vi "ao_waveform_full.vi"() -> ()   [LabVIEW 2020]
uses:
  <vilib>/measure/NI_MABase.lvlib
panel:
  in  "Offset":dbl
  in  "signal type":T1(ring) caption="Signal Type"
  out "error out":errorcluster caption="错误输出"
  in  "Frequency":dbl=1000.0 format="%#.6g"
  in  "Amplitude":dbl=5.0 format="%.3f"
  out "波形图":waveform(dbl)(graph)
  in  "AoCycle":u32
  in  "SamplePeriod(ns)":u32=10000
  in  "Chan":u8
  in  "DevIndex":i32
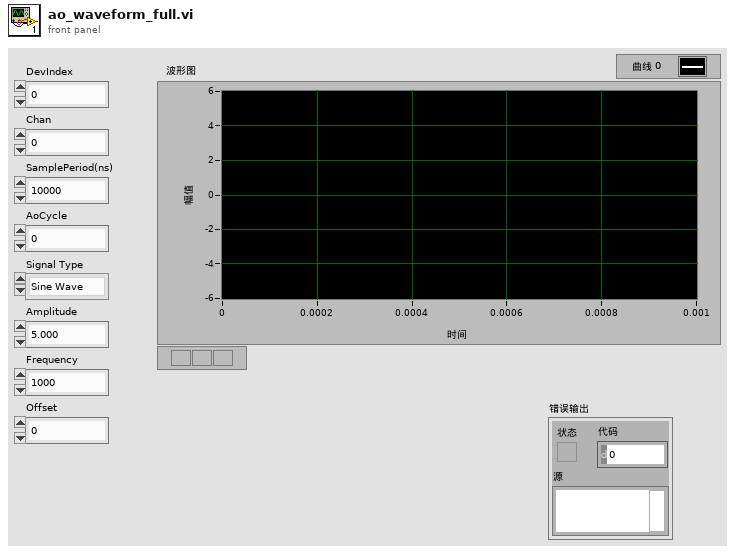
[diagram p1: front panel]
types:
  T1 = enum16{"Sine Wave", "Triangle Wave", "Square Wave", "Sawtooth Wave"}
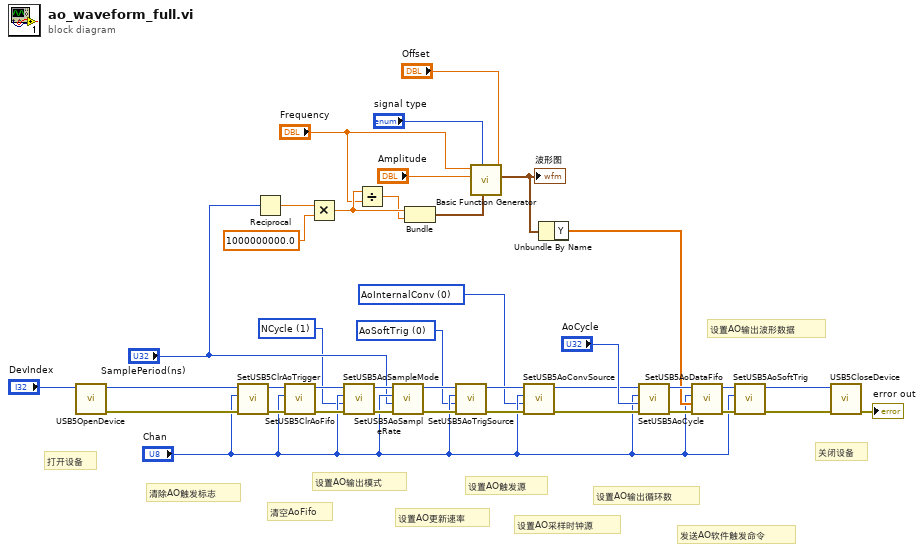
[diagram p0: block diagram]
diagram:
  w1 = u8 0 items=["AoInternalConv", "ConvIn", "AiConv", "DiConv", "DoConv", "Ao0Conv", "Ao1Conv", "Ao2Conv", "Ao3Conv"] ("AoConvSource")
  w2 = u8 0 items=["AoSoftTrig"=0, "ExtTrigIn"=1, "Din0RisingEdge"=2, "Din1RisingEdge"=3, "Din2RisingEdge"=4, "Din3RisingEdge"=5, "WithAiTrig"=6, "WithDiTrig"=7, "WithDoTrig"=8, "WithAo0Trig"=9, "WithAo1Trig"=10, "WithAo2Trig"=11, "WithAo3Trig"=12, "GlobalSoftTrig"=255] ("AoTrigSource")
  w3 = u8 1 items=["PcBufferedInfinite", "NCycle"] ("SampleMode")
  # "关闭设备"
  # "发送AO软件触发命令"
  # "设置AO输出波形数据"
  # "设置AO输出循环数"
  # "设置AO采样时钟源"
  # "设置AO触发源"
  # "设置AO更新速率"
  # "设置AO输出模式"
  # "清空AoFifo"
  # "清除AO触发标志"
  # "打开设备"
  n1 = call "USB5OpenDevice.vi"("DevIndex"="DevIndex") -> ("error out"=w20:errorcluster, "DevIndex Out"=w17:i32)  [unwired: 9 in]
  n2 = call "SetUSB5ClrAoTrigger.vi"("错误输入（无错误）"=w20, "Chan"="Chan", "DevIndex"=w17) -> ("错误输出"=w19:errorcluster, "DevIndex Out"=w18:i32)  [unwired: 7 in]
  n3 = Reciprocal(x="SamplePeriod(ns)") -> (1/x=w39:dbl)
  n4 = call "SetUSB5ClrAoFifo.vi"("错误输入（无错误）"=w19, "Chan"="Chan", "DevIndex"=w18) -> ("错误输出"=w15:errorcluster, "DevIndex Out"=w16:i32)  [unwired: 7 in]
  n5 = Multiply(x=w39, y=1000000000.0) -> (x*y=w36:dbl)
  n6 = call "SetUSB5AoSampleMode.vi"("错误输入（无错误）"=w15, "SampleMode"=w3, "Chan"="Chan", "DevIndex"=w16) -> ("错误输出"=w14:errorcluster, "DevIndex Out"=w13:i32)  [unwired: 6 in]
  n7 = Divide(x=w36, y="Frequency") -> (x/y=w5:dbl)
  n8 = call "SetUSB5AoSampleRate.vi"("错误输入（无错误）"=w14, "SamplePeriod(ns)"="SamplePeriod(ns)", "Chan"="Chan", "DevIndex"=w13) -> ("错误输出"=w11:errorcluster, "DevIndex Out"=w12:i32)  [unwired: 6 in]
  n9 = Bundle(w36, w5) -> (w38:cluster{dbl, dbl})  [unwired: 1 in]
  n10 = call "SetUSB5AoTrigSource.vi"("错误输入（无错误）"=w11, "AoTrigSource"=w2, "Chan"="Chan", "DevIndex"=w12) -> ("错误输出"=w9:errorcluster, "DevIndex Out"=w10:i32)  [unwired: 6 in]
  n11 = call <vilib>:"Basic Function Generator.vi"("offset"="Offset", "sampling info"=w38, "signal type"="signal type", "amplitude"="Amplitude", "frequency"="Frequency") -> ("signal out"=w24:waveform(dbl))  [unwired: 4 in, 2 out]
  "波形图" <- w24
  n12 = call "SetUSB5AoConvSource.vi"("错误输入（无错误）"=w9, "AoConvSource"=w1, "Chan"="Chan", "DevIndex"=w10) -> ("错误输出"=w7:errorcluster, "DevIndex Out"=w8:i32)  [unwired: 6 in]
  n13 = Unbundle By Name(w24) -> ("Y"=w23:dbl[])
  n14 = call "SetUSB5AoCycle.vi"("错误输入（无错误）"=w7, "AoCycle"="AoCycle", "Chan"="Chan", "DevIndex"=w8) -> ("错误输出"=w31:errorcluster, "DevIndex Out"=w30:i32)  [unwired: 6 in]
  n15 = call "SetUSB5AoDataFifo.vi"("错误输入（无错误）"=w31, "Voltage"=w23, "Chan"="Chan", "DevIndex"=w30) -> ("错误输出"=w28:errorcluster, "DevIndex Out"=w29:i32)  [unwired: 6 in]
  n16 = call "SetUSB5AoSoftTrig.vi"("错误输入（无错误）"=w28, "Chan"="Chan", "DevIndex"=w29) -> ("错误输出"=w26:errorcluster, "DevIndex Out"=w27:i32)  [unwired: 7 in]
  n17 = call "USB5CloseDevice.vi"("错误输入（无错误）"=w26, "DevIndex"=w27) -> ("error out"=→"error out":errorcluster)  [unwired: 8 in, 1 out]
